vi "intRandom.vi"() -> ()   [LabVIEW 2011, in "IntClass.lvclass"]
uses:
  IntClass.lvclass
  UintClass/enumBase.ctl
  IntClass.lvclass/IntClass.ctl
  <userlib>/_OpenG.lib/numeric/numeric.llb/Random Number Within Range - I32__ogtk.vi
  UintClass/UintClass.lvclass
panel:
  out "Error out":errorcluster
  out "Int out":refnum<class "IntClass.lvclass">
  in  "Negative":bool=TRUE
  in  "Error in (no error)":errorcluster
  in  "Base (decimal)":T1=10 items=["Binary"=2, "Octal"=8, "Decimal"=10, "Hexadecimal"=16, "Hexatrigesimal"=36, "ASCII"=64]
  in  "Number of decimals":i32=100
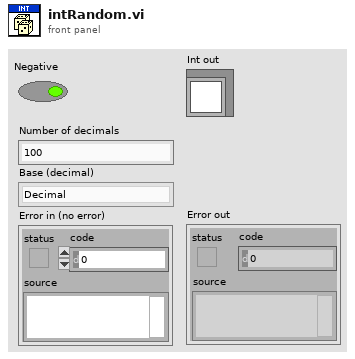
[diagram p1: front panel]
types:
  T1 = typedef "UintClass.lvclass/enumBase.ctl" = u16
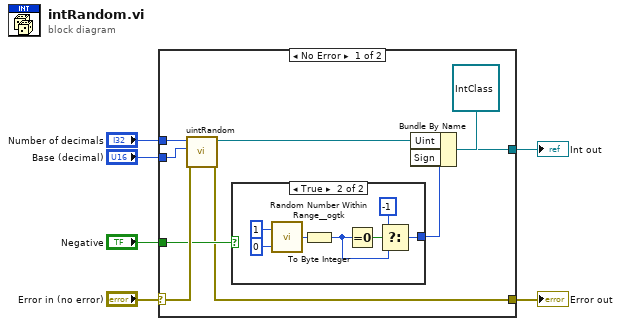
[diagram p0: block diagram]
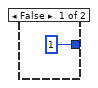
[diagram p2: hidden frame]
diagram:
  n1 = case shown="No Error" "Error in (no error)" {
    selector: "Error in (no error)" -> [w13 w24]
    tunnel: "Number of decimals" -> [w15 _]
    tunnel: "Base (decimal)" -> [w14 _]
    tunnel: "Negative" -> [w12 _]
    tunnel: [w8 w24] -> w2
    tunnel: [w7 _] -> w1
    frame No Error {
      n2 = call "uintRandom.vi"("Error in (no error)"=w13, "Base (decimal)"=w14, "Number of decimals"=w15) -> ("Error out"=w8:errorcluster, "Uint out"=w11:refnum<class "UintClass.lvclass">)  [unwired: 7 in]
      n3 = case shown="True" w12 {
        tunnel: [i8 1 w19] -> w9
        frame False {
        }
        frame True {
          n4 = call-poly <userlib>:"Random Number Within Range__ogtk.vi"("High"=1, "Low"=0) -> ("Random Number"=w21:i32)  [unwired: 3 in]
          n5 = To Byte Integer(number=w21) -> (8bit integer=w18:i8)
          n6 = Equal To 0?(x=w18) -> (x = 0?=w20:bool)
          n7 = Select(t=i8 -1, s=w20, f=w18) -> (s? t:f=w19:i8)
        }
      }
      n8 = Bundle By Name(cluster=refnum<class "IntClass.lvclass"> refnum ("Int out"), "Uint"=w11, "Sign"=w9) -> (w7:refnum<class "IntClass.lvclass">)
    }
    frame Error {
    }
  }
  "Int out" <- w1
  "Error out" <- w2
